vi "pp_genStimList.vi"(0 "Total Trials":i32=12 min=2, 5 "Go Stims":dbl[][](array[numeric])=[[1.0, 2.0, 3.0, 0.0, 0.0, 0.0], [2.0, 3.0, 4.0, 0.0, 0.0, 0.0], [3.0, 4.0, 5.0, 0.0, 0.0, 0.0]], 7 "NoGo Stims":dbl[][](array[numeric])=[[5.0, 6.0, 7.0, 0.0, 0.0, 0.0, 5.0], [6.0, 7.0, 8.0, 0.0, 0.0, 0.0, 0.0], [7.0, 8.0, 9.0, 0.0, 0.0, 0.0, 0.0]], 11 "error in (no error)":errorcluster) -> (4 "Session Stim List":dbl[][](array[numeric])=[[1.0, 2.0, 3.0, 4.0, 0.0, 0.0, 0.0, 0.0], [1.0, 3.0, 4.0, 5.0, 0.0, 0.0, 0.0, 0.0], [1.0, 1.0, 2.0, 3.0, 0.0, 0.0, 0.0, 0.0], [0.0, 7.0, 8.0, 9.0, 0.0, 0.0, 0.0, 0.0], [1.0, 2.0, 3.0, 4.0, 0.0, 0.0, 0.0, 0.0], [0.0, 7.0, 8.0, 9.0, 0.0, 0.0, 0.0, 0.0], [0.0, 5.0, 6.0, 7.0, 0.0, 0.0, 0.0, 5.0], [1.0, 3.0, 4.0, 5.0, 0.0, 0.0, 0.0, 0.0], [0.0, 6.0, 7.0, 8.0, 0.0, 0.0, 0.0, 0.0], [1.0, 1.0, 2.0, 3.0, 0.0, 0.0, 0.0, 0.0], [0.0, 5.0, 6.0, 7.0, 0.0, 0.0, 0.0, 5.0], [0.0, 6.0, 7.0, 8.0, 0.0, 0.0, 0.0, 0.0]], 15 "error out":errorcluster)   [LabVIEW 2013]
uses:
  labolabo/array/impl/PrependRows_D.vi
panel:
  # "Stim Code, Stim Type, Duration, Param 1, Param 2, Param 3, Param 4"
  # "Stim Code, Stim Type, Duration, Param 1, Param 2, Param 3, Param 4"
  # "GONOGO, Stim Code, Stim Type, Duration, Param 1, Param 2, Param 3, Param 4"
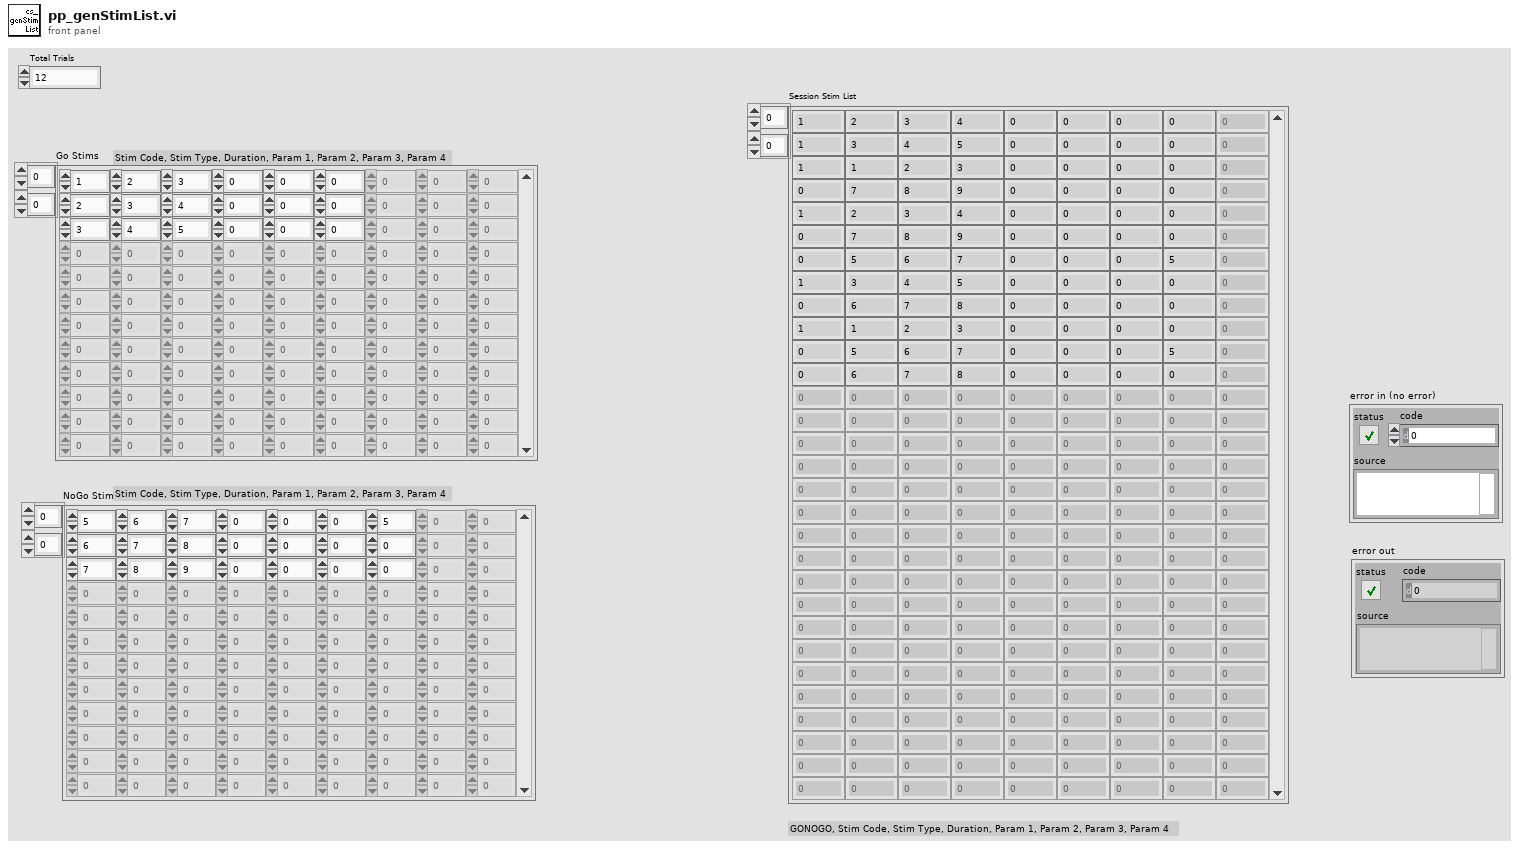
[diagram p1: front panel]
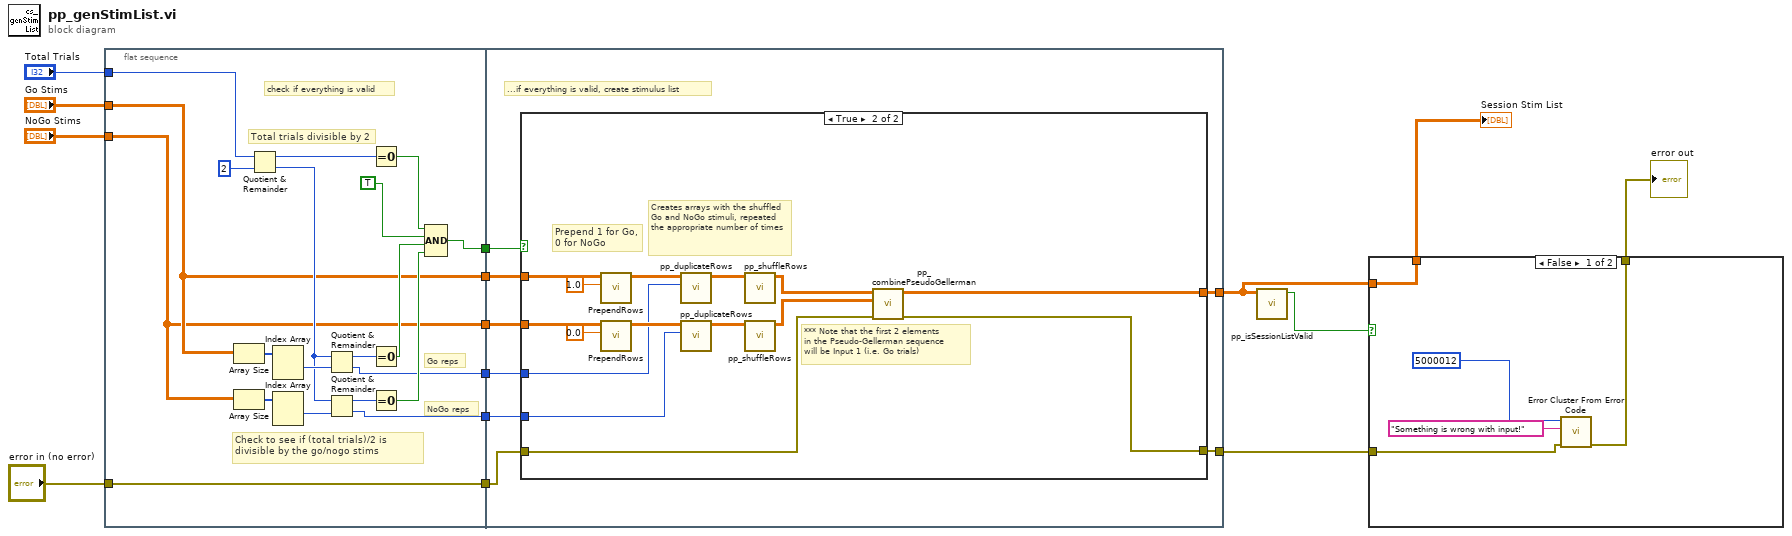
[diagram p0: block diagram]
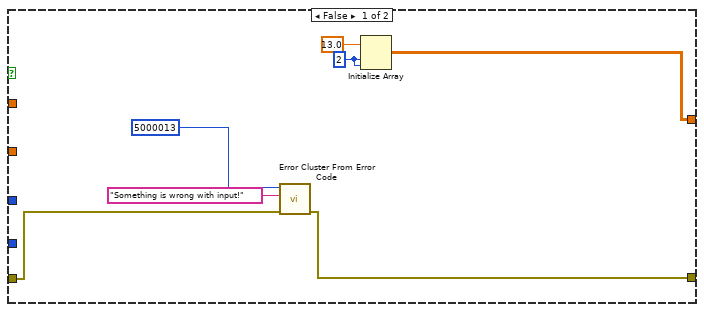
[diagram p3: hidden frame]
diagram:
  n1 = flat-sequence {
    tunnel: "Go Stims" -> [w18]
    tunnel: "NoGo Stims" -> [w17]
    tunnel: "Total Trials" -> [w22]
    tunnel: [w21] -> w12
    tunnel: [w20] -> w11
    tunnel: [w19] -> w10
    tunnel: [w18] -> w9
    tunnel: [w17] -> w8
    tunnel: [w16] -> w4
    tunnel: "error in (no error)" -> [w16]
    tunnel: w12 -> [w43]
    tunnel: w11 -> [w42]
    tunnel: w10 -> [w41]
    tunnel: w9 -> [w40]
    tunnel: w8 -> [w39]
    tunnel: [w38] -> w6
    tunnel: w4 -> [w37]
    tunnel: [w36] -> w2
    frame #0 {
      # "NoGo reps"
      # "Go reps"
      # "check if everything is valid"
      # "Check to see if (total trials)/2 is divisible by the go/nogo stims"
      # "Total trials divisible by 2"
      n2 = Array Size(array=w18) -> (size(s)=w23:i32[])
      n3 = Array Size(array=w17) -> (size(s)=w24:i32[])
      n4 = Quotient & Remainder(x=w22, y=2) -> (x-y*floor(x/y)=w27:i32, floor(x/y)=w26:i32)
      n5 = Index Array(array=w23) -> (element #1=w33:i32)  [unwired: 2 in, 1 out]
      n6 = Index Array(array=w24) -> (element #1=w34:i32)  [unwired: 2 in, 1 out]
      n7 = Quotient & Remainder(x=w26, y=w33) -> (x-y*floor(x/y)=w29:i32, floor(x/y)=w20:i32)
      n8 = Quotient & Remainder(x=w26, y=w34) -> (x-y*floor(x/y)=w30:i32, floor(x/y)=w19:i32)
      n9 = Equal To 0?(x=w27) -> (x = 0?=w28:bool)
      n10 = Equal To 0?(x=w29) -> (x = 0?=w31:bool)
      n11 = Equal To 0?(x=w30) -> (x = 0?=w32:bool)
      n12 = Compound Arithmetic op=AND(w28, TRUE, w31, w32) -> (w21:bool)
    }
    frame #1 {
      # "...if everything is valid, create stimulus list"
      n13 = case shown="True" w43 {
        tunnel: w42 -> [_ w59]
        tunnel: w41 -> [_ w58]
        tunnel: w40 -> [_ w65]
        tunnel: w39 -> [_ w62]
        tunnel: [w50 w53] -> w38
        tunnel: w37 -> [w45 w52]
        tunnel: [w44 w51] -> w36
        frame False {
          w48 = 2 ("dimension size")
          n14 = call <vilib>:"Error Cluster From Error Code.vi"("error in (no error)"=w45, "error message (\"\")"="Something is wrong with input!" ("error message (\"\")"), "error code (0)"=5000013) -> ("error out"=w44:errorcluster)  [unwired: 6 in]
          n15 = Initialize Array(13.0 ("element"), w48, w48) -> (w50:dbl[][])
        }
        frame True {
          # "*** Note that the first 2 elements\nin the Pseudo-Gellerman sequence\nwill be Input 1 (i.e. Go trials)"
          # "Prepend 1 for Go,\n0 for NoGo"
          # "Creates arrays with the shuffled Go and NoGo stimuli, repeated the appropriate number of times"
          n16 = call-poly "PrependRows.vi"("Prepend Value"=1.0, "Input"=w65) -> ("Output"=w61:dbl[][])  [unwired: 9 in]
          n17 = call-poly "PrependRows.vi"("Prepend Value"=0.0, "Input"=w62) -> ("Output"=w60:dbl[][])  [unwired: 9 in]
          n18 = call "pp_duplicateRows.vi"("Repetitions"=w59, "Input"=w61) -> ("Output"=w57:dbl[][])  [unwired: 9 in]
          n19 = call "pp_duplicateRows.vi"("Repetitions"=w58, "Input"=w60) -> ("Output"=w56:dbl[][])  [unwired: 9 in]
          n20 = call "pp_shuffleRows.vi"("Input"=w57) -> ("Output"=w55:dbl[][])  [unwired: 10 in]
          n21 = call "pp_shuffleRows.vi"("Input"=w56) -> ("Output"=w54:dbl[][])  [unwired: 10 in]
          n22 = call "pp_combinePseudoGellerman.vi"("error in (no error)"=w52, "Input2"=w54, "Input1"=w55) -> ("error out"=w51:errorcluster, "Output"=w53:dbl[][])  [unwired: 7 in]
        }
      }
    }
  }
  n23 = call "pp_isSessionListValid.vi"("Array"=w6) -> ("Valid?"=w7:bool)  [unwired: 9 in, 1 out]
  n24 = case shown="False" w7 {
    tunnel: w6 -> [w66 w72]
    tunnel: [w66 w72] -> w5
    tunnel: w2 -> [w68 w71]
    tunnel: [w67 w71] -> w1
    frame False {
      n25 = call <vilib>:"Error Cluster From Error Code.vi"("error in (no error)"=w68, "error message (\"\")"="Something is wrong with input!" ("error message (\"\")"), "error code (0)"=5000012) -> ("error out"=w67:errorcluster)  [unwired: 6 in]
    }
    frame True {
    }
  }
  "Session Stim List" <- w5
  "error out" <- w1
